vi "Stop Core.vi"(10 "final error code":i32, 11 "Base UI Component in":refnum<class "Base UI Component.lvclass">) -> (3 "Base UI Component out":refnum<class "Base UI Component.lvclass">)   [LabVIEW 2016, in "Assert Display.lvlib" / "Base UI Component.lvlib" / "Base UI Component.lvclass"]
doc: "(<B>Filename</B>: Actor Framework.lvlib:Actor.lvclass:Stop Core.vi)\n\nDefines what the actor does before it stops. Use the <B>final error code</B> input to determine whether the actor shut down in response to an error.\n\nBy default, this method does nothing. A descendant class may override it to define behavior, such as shutting down any processes the actor initiated in its override of the Actor Core method."
uses:
  Base UI Component.lvclass
  Base UI Component.lvclass/Base UI Component.ctl
  Base UI Actor/Base UI Actor/Base UI Actor.lvclass
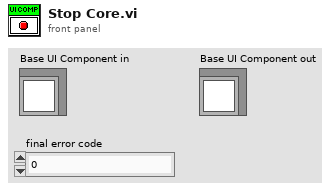
[diagram p1: front panel]
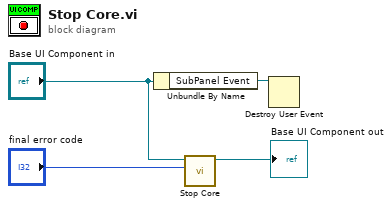
[diagram p0: block diagram]
diagram:
  n1 = Unbundle By Name("Base UI Component in") -> ("SubPanel Event"=w2:refnum<user-event>)
  n2 = call-parent "Stop Core.vi"("final error code"="final error code", "Base UI Actor in"="Base UI Component in") -> ("Base UI Actor out"=→"Base UI Component out":refnum<class "Base UI Component.lvclass">)  [unwired: 9 in]
  n3 = Destroy User Event(user event=w2) -> ()  [unwired: 1 in, 1 out]
